vi "Test_ReadValue_TransportClosed_ReadError.vi"(8 "error in (no error)":errorcluster, 11 "TestCase in":refnum<class "TestNotifierTransport.lvclass">) -> (0 "error out":errorcluster, 3 "TestCase out":refnum<class "TestNotifierTransport.lvclass">)   [LabVIEW 2017, in "TestNotifierTransport.lvclass"]
uses:
  TestNotifierTransport.lvclass
  Source/Concrete/NotifierTransport/NotifierTransport.lvclass/NotifierTransport.ctl
  <vilib>/Utility/error.llb/Error Cluster From Error Code.vi
  Source/Concrete/NotifierTransport/NotifierTransport.lvclass
panel:
  out "Return Error":errorcluster
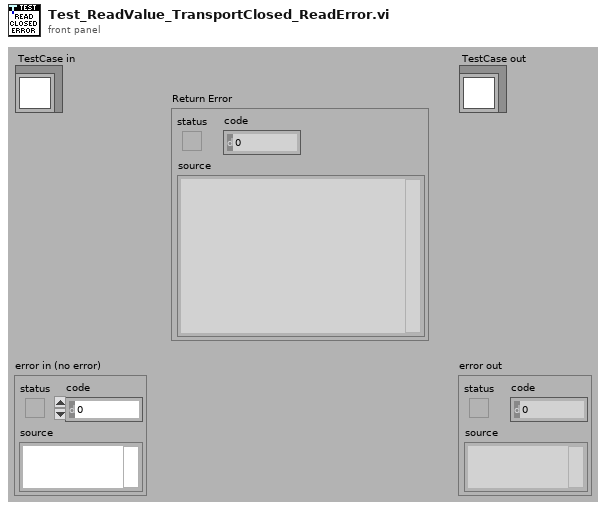
[diagram p1: front panel]
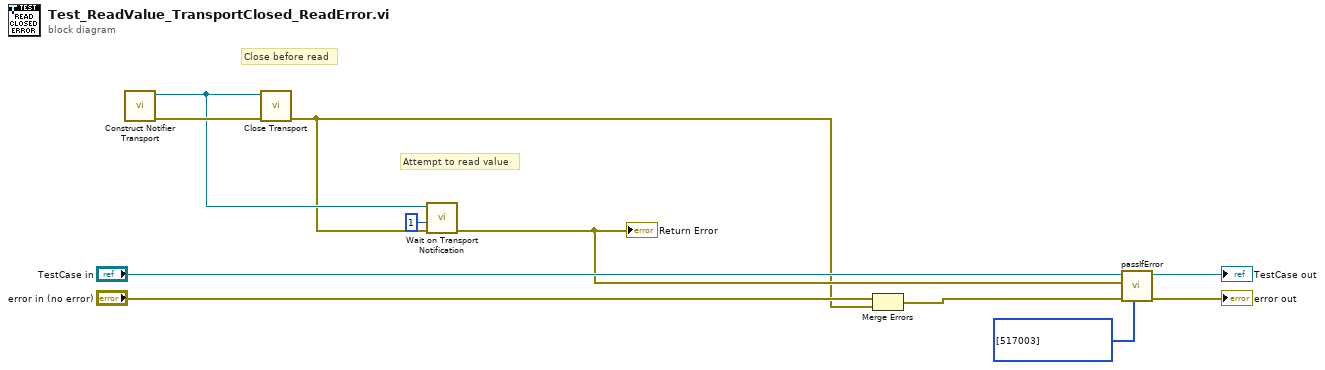
[diagram p0: block diagram]
diagram:
  # "Close before read"
  # "Attempt to read value"
  n1 = call "Construct Notifier Transport.vi"() -> ("error out"=w4:errorcluster, "NotifierTransport"=w2:refnum<class "NotifierTransport.lvclass">)  [unwired: 10 in]
  n2 = call-dynamic "Close Transport.vi"("error in (no error)"=w4, "NotifierTransport"=w2) -> ("error out"=w1:errorcluster)  [unwired: 9 in]
  n3 = call "Wait on Transport Notification.vi"("error in (no error)"=w1, "Timeout In ms (-1)"=1, "NotifierTransport"=w2) -> ("error out"=w3:errorcluster)  [unwired: 6 in, 2 out]
  "Return Error" <- w3
  n4 = Merge Errors("error in (no error)", w1) -> (w6:errorcluster)
  n5 = call-dynamic "passIfError.vi"("passing error codes (default = any error code)"=i32[] [517003], "error in (no error)"=w6, "error"=w3, "TestCase in"="TestCase in") -> ("error out"=→"error out":errorcluster, "TestCase out"=→"TestCase out":refnum<class "TestNotifierTransport.lvclass">)  [unwired: 6 in]
